vi "PanelMsg (SubVI).vi"(0 "String in":refnum<vi>, 2 "Error?(T)":bool, 3 "ErrorMsg":string, 4 "OKMsg":string, 5 "error in (no error)":errorcluster) -> (19 "error out":errorcluster)   [LabVIEW 2017]
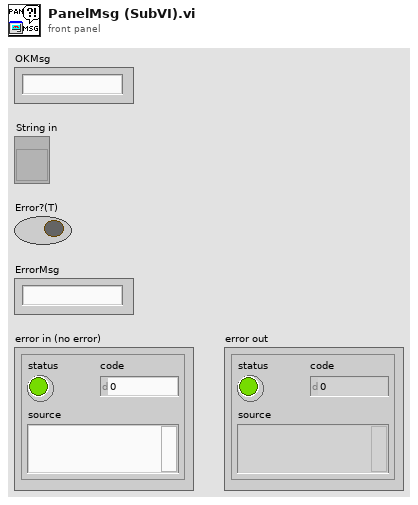
[diagram p1: front panel]
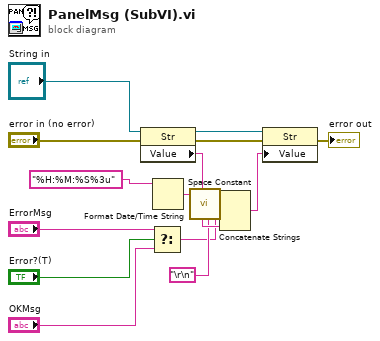
[diagram p0: block diagram]
diagram:
  n1 = property class="Str"(reference="String in", error in="error in (no error)") -> (reference out=w6:refnum<vi>, error out=w11:errorcluster, "Value"=w4:string)
  n2 = Select(t="ErrorMsg", s="Error?(T)", f="OKMsg") -> (s? t:f=w2:string)
  n3 = Format Date/Time String(time format string (%c)="%H:%M:%S%3u") -> (date/time string=w8:string)  [unwired: 2 in]
  n4 = call <vilib>:"Space Constant.vi"() -> ("String"=w1:string)
  n5 = Concatenate Strings(w8, w1, w2, "\r\n", w4) -> (w9:string)
  n6 = property class="Str"(reference=w6, error in=w11, "Value"=w9) -> (error out=→"error out":errorcluster)  [unwired: 1 out]
